vi "CreatePriorityQueue.vi"(8 "error in (no error)":errorcluster) -> (0 "error out":errorcluster, 3 "PriorityQueue":refnum<data-value>)   [LabVIEW 2009, in "PriorityQueue.lvlib"]
uses:
  PriorityQueue.lvlib
  PriorityQueue/PriorityQueue.lvclass
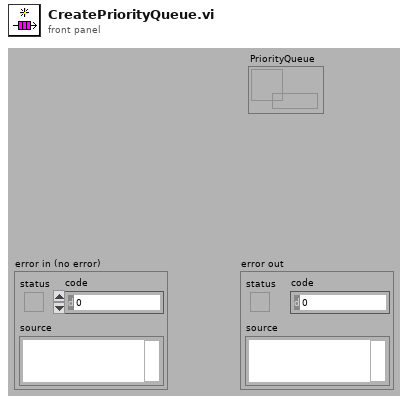
[diagram p1: front panel]
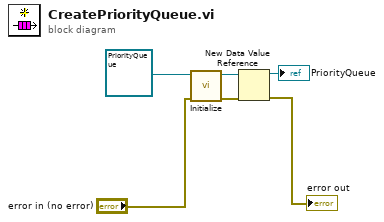
[diagram p0: block diagram]
diagram:
  n1 = call-dynamic "Initialize.vi"("error in (no error)"="error in (no error)", "PriorityQueue in"=refnum<class "PriorityQueue.lvclass"> refnum ("PriorityQueue.lvclass")) -> ("error out"=w2:errorcluster, "PriorityQueue out"=w5:refnum<class "PriorityQueue.lvclass">)  [unwired: 8 in]
  n2 = New Data Value Reference(data value=w5, error in=w2) -> (data value reference=→"PriorityQueue":refnum<data-value>, error out=→"error out":errorcluster)
